vi "Get Temperature Reading.vi"(0 "Session Handle in":T1, 11 "error in (no error)":errorcluster) -> (4 "Session Handle out":T1, 6 "Failure Reason":string, 8 "Success?":bool, 10 "Temperature":dbl, 15 "error out":errorcluster)   [LabVIEW 2015, in "Oil.lvclass"]
uses:
  Oil.lvclass
  Typedefs/Session Handle.ctl
panel:
  in  "Temp Sensor":u8=25 format="%x"
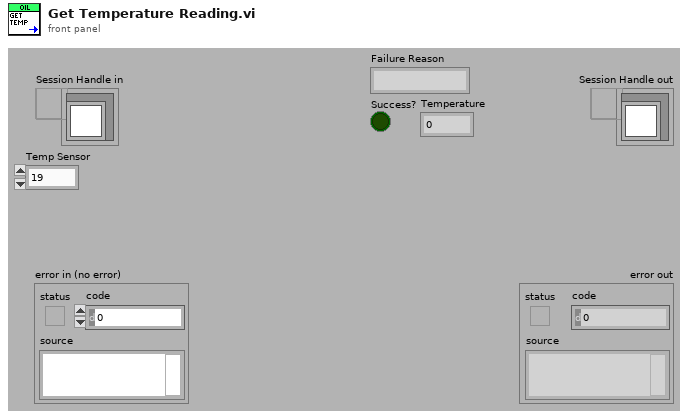
[diagram p1: front panel]
types:
  T1 = typedef "Oil.lvclass/Session Handle.ctl" = refnum<data-value>
  T2 = typedef "XNET Frame CAN.ctl" = cluster{"timestamp":timestamp, "payload":u8[], "identifier":u32, "type":T3, "extended?":bool, "echo?":bool}
  T3 = typedef "XNET Frame Type CAN.ctl" = u8
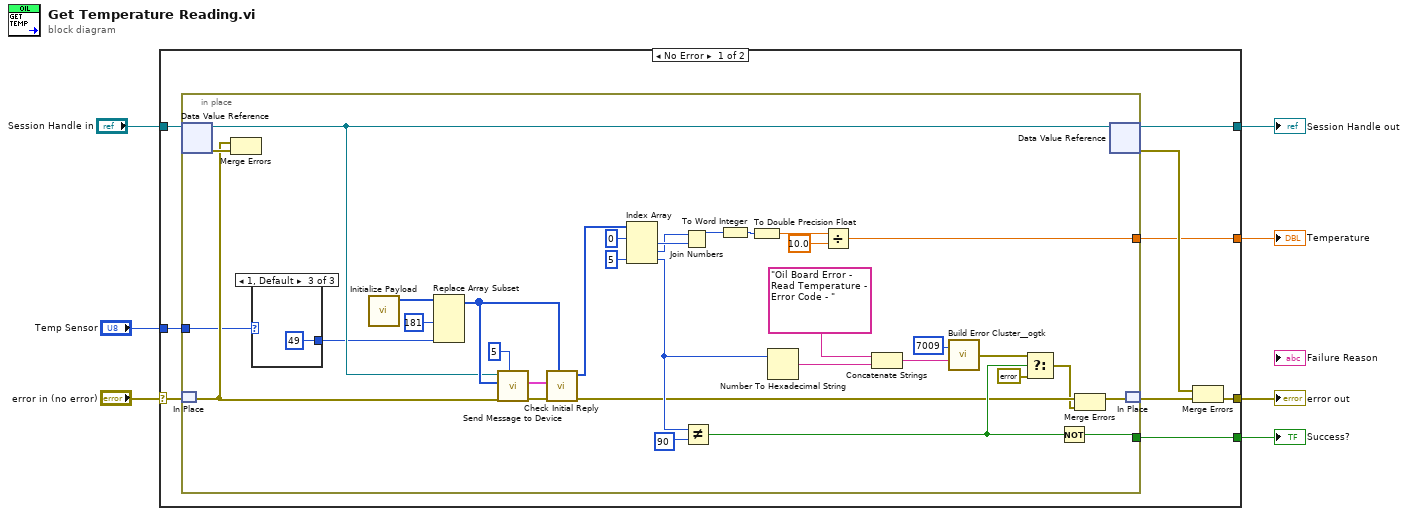
[diagram p0: block diagram]
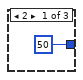
[diagram p2: hidden frame]
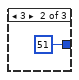
[diagram p3: hidden frame]
diagram:
  n1 = case shown="No Error" "error in (no error)" {
    selector: "error in (no error)" -> [w11 w54]
    tunnel: "Session Handle in" -> [w16 w55]
    tunnel: [w15 w55] -> w6
    tunnel: [w12 w54] -> w5
    tunnel: [w10 _] -> w3
    tunnel: [w9 _] -> w2
    tunnel: "Temp Sensor" -> [w8 _]
    frame No Error {
      n2 = in-place {
        in-place-border: [w25] -> w10
        in-place-border: [w35] -> w9
        in-place-border: w8 -> [w34]
        n3 = in-place-dvr #1(w16) -> (w43:refnum<class "Oil.lvclass">, w50:errorcluster)
        n4 = in-place-match #2(w11) -> (w44:errorcluster)
        n5 = Merge Errors(w44, w50) -> ()  [unwired: 1 out]
        n6 = case shown="1, Default" w34 {
          tunnel: [u8 50 ("new element/subarray") u8 51 ("new element/subarray") u8 49 ("new element/subarray")] -> w33
          frame 2 {
          }
          frame 3 {
          }
          frame 1, Default {
          }
        }
        n7 = call "Initialize Payload.vi"() -> ("Initial Payload"=w49:u8[])  [unwired: 11 in]
        n8 = Replace Array Subset(array=w49, new element #1=u8 181 ("new element/subarray"), new element #2=w33) -> (w45:u8[])  [unwired: 2 in]
        n9 = call "Send Message to Device.vi"("Number of Retries"=5, "error in (no error)"=w44, "payload"=w45, "CAN Comm In"=w43) -> ("error out"=w26:errorcluster, "Reply"=w46:T2[])  [unwired: 5 in, 1 out]
        n10 = call "Check Initial Reply.vi"("Write Message"=w45, "error in (no error)"=w26, "Reply"=w46) -> ("error out"=w20:errorcluster, "Data Packet 2"=w42:u8[])  [unwired: 5 in, 2 out]
        n11 = Index Array(array=w42, index #1=0 ("index"), index #3=5 ("index")) -> (element #1=w41:u8, element #2=w40:u8, element #3=w30:u8)  [unwired: 1 in]
        n12 = Join Numbers(hi=w40, lo=w41) -> ((hi.lo)=w29:u16)
        n13 = Not Equal?(x=w30, y=u8 90 ("new element/subarray")) -> (x != y?=w21:bool)
        n14 = To Word Integer(number=w29) -> (16bit integer=w28:i16)
        n15 = To Double Precision Float(number=w28) -> (double precision float=w27:dbl)
        n16 = Number To Hexadecimal String(2:w30) -> (0:w36:string)  [unwired: 1 in]
        n17 = Divide(x=w27, y=10.0) -> (x/y=w35:dbl)
        n18 = Concatenate Strings("Oil Board Error - Read Temperature - Error Code - ", w36) -> (w24:string)
        n19 = call <userlib>:"Build Error Cluster__ogtk.vi"("String to Prepend to source (\"\")"=w24, "code"=7009) -> ("error out"=w23:errorcluster)
        n20 = Select(t=w23, s=w21, f=errorcluster {"status"=FALSE, "code"=0, "source"=""}) -> (s? t:f=w19:errorcluster)
        n21 = Not(x=w21) -> (.not. x?=w25:bool)
        n22 = Merge Errors(w20, w19) -> (w18:errorcluster)
        n23 = in-place-dvr #1(w43) -> (w15:T1, w13:errorcluster)
        n24 = in-place-match #2(w18) -> (w14:errorcluster)
      }
      n25 = Merge Errors(w13, w14) -> (w12:errorcluster)
    }
    frame Error {
    }
  }
  "Session Handle out" <- w6
  "error out" <- w5
  "Success?" <- w3
  "Temperature" <- w2
